vi "Power Output Execute Measurement.vi"(0 "Plots":T15, 1 "Measurement Data In":T11[](array[typedef]), 2 "TestSetDef":T1={"General"={"ID"=0, "Model"="", "Dual Port?"=FALSE, "Options"="", "Options"={"E"=FALSE, "K"=FALSE, "H"=FALSE, "W"=FALSE, "F"=FALSE}, "Cal File"=path ""}, "Receiver"={"Fstart, MHz"=0.0, "Fstop MHz"=0.0, "Fstep MHz"=0.0, "IF, MHz"=0.0}, "RX Band"={"Fstart, MHz"=0.0, "Fstop MHz"=0.0}, "TX 1"={"Fstart, MHz"=0.0, "Fstop MHz"=0.0, "Pmax, dBm"=0.0, "Pstep, dB"=0.0}, "TX 2"={"Fstart, MHz"=0.0, "Fstop MHz"=0.0, "Pmax, dBm"=0.0, "Pstep, dB"=0.0}, "Low-side?"=TRUE}, 3 "Queue":refnum<queue>, 5 "Test Parameters":T2={"Stimulus"={"Frequency Type"=enum."Band Edges", "Frequency Ranges"=[], "TX 1 Frequency (MHz)"={"Min"=0.0, "Max"=0.0}, "TX 2 Frequency (MHz)"={"Min"=0.0, "Max"=0.0}, "RX Frequency (MHz)"={"Min"=0.0, "Max"=0.0}, "Pad Model Number"="", "Pad Serial Number"="", "Pad Values"=[]}, "Measurement"={"DUT Port"=enum."Port 1", "Direction"=0, "Frequency Step Size"=0}, "Display"={"Frequency"={"Min"=-1.0, "Max"=-1.0}, "Power"={"Min"=-1, "Max"=-1}}, "Limit"={"Min Power (dBm)"=44.0}, "Calibration"={"Calibrated?"=FALSE}} {"Measurement"."Frequency Step Size" items=["0.2", "0.4", "1.0", "2.0", "4.0"]; "Measurement"."Direction" items=["Reverse", "Forward", "Auxiliary"]}, 9 "Measured Values":refnum<vi>, 11 "error in (no error)":errorcluster, 12 "Driver Refs In":T14, 13 "Measurements":refnum<vi>) -> (4 "Pass/Fail":bool[](array[boolean]), 6 "Test Parameters Out":T2={"Stimulus"={"Frequency Type"=enum."Band Edges", "Frequency Ranges"=[], "TX 1 Frequency (MHz)"={"Min"=0.0, "Max"=0.0}, "TX 2 Frequency (MHz)"={"Min"=0.0, "Max"=0.0}, "RX Frequency (MHz)"={"Min"=0.0, "Max"=0.0}, "Pad Model Number"="", "Pad Serial Number"="", "Pad Values"=[]}, "Measurement"={"DUT Port"=enum."Port 1", "Direction"=0, "Frequency Step Size"=0}, "Display"={"Frequency"={"Min"=-1.0, "Max"=-1.0}, "Power"={"Min"=-1, "Max"=-1}}, "Limit"={"Min Power (dBm)"=44.0}, "Calibration"={"Calibrated?"=FALSE}} {"Measurement"."Frequency Step Size" items=["0.2", "0.4", "1.0", "2.0", "4.0"]; "Measurement"."Direction" items=["Reverse", "Forward", "Auxiliary"]}, 10 "Measurement Data Out":T11[](array[typedef]), 14 "Driver Refs Out":T14, 15 "error out":errorcluster)   [LabVIEW 2011]
uses:
  TypeDefs/Power Output Test Parameters.ctl
  TypeDefs/Power Output Stimulus Parameters.ctl
  TypeDefs/Power Output Measurement Parameters.ctl
  BPIMCore EXT/HW IO/DUTport.ctl
  BPIMCore EXT/HW IO/MeasMode.ctl
  BPIMCore EXT/HW IO/PIM Sweep Step Size.ctl
  TypeDefs/Power Output Display Parameters.ctl
  TypeDefs/Power Output Limit Parameters.ctl
  TypeDefs/Power Output Calibration State.ctl
  drivers/PIM/PIM Driver Ref.ctl
  drivers/PWM/PWM Driver Ref.ctl
  TypeDefs/Power Output Measurement Data.ctl
  TypeDefs/Power Output Queue Cluster.ctl
  BPIMCore EXT/HW IO/Test Set Definition.ctl
  drivers/PIM/PIM Command.ctl
  Summitek EXT/Miscellaneous/OGAB Version.ctl
  drivers/PWM/PWM Parameters.ctl
  drivers/PWM/PWM Command.ctl
  Summitek EXT/OpenG EXT/array/array.llb/Remove Duplicates from 1D Array (DBL)__ogtk.vi
  <vilib>/Analysis/NI_AALBase.lvlib
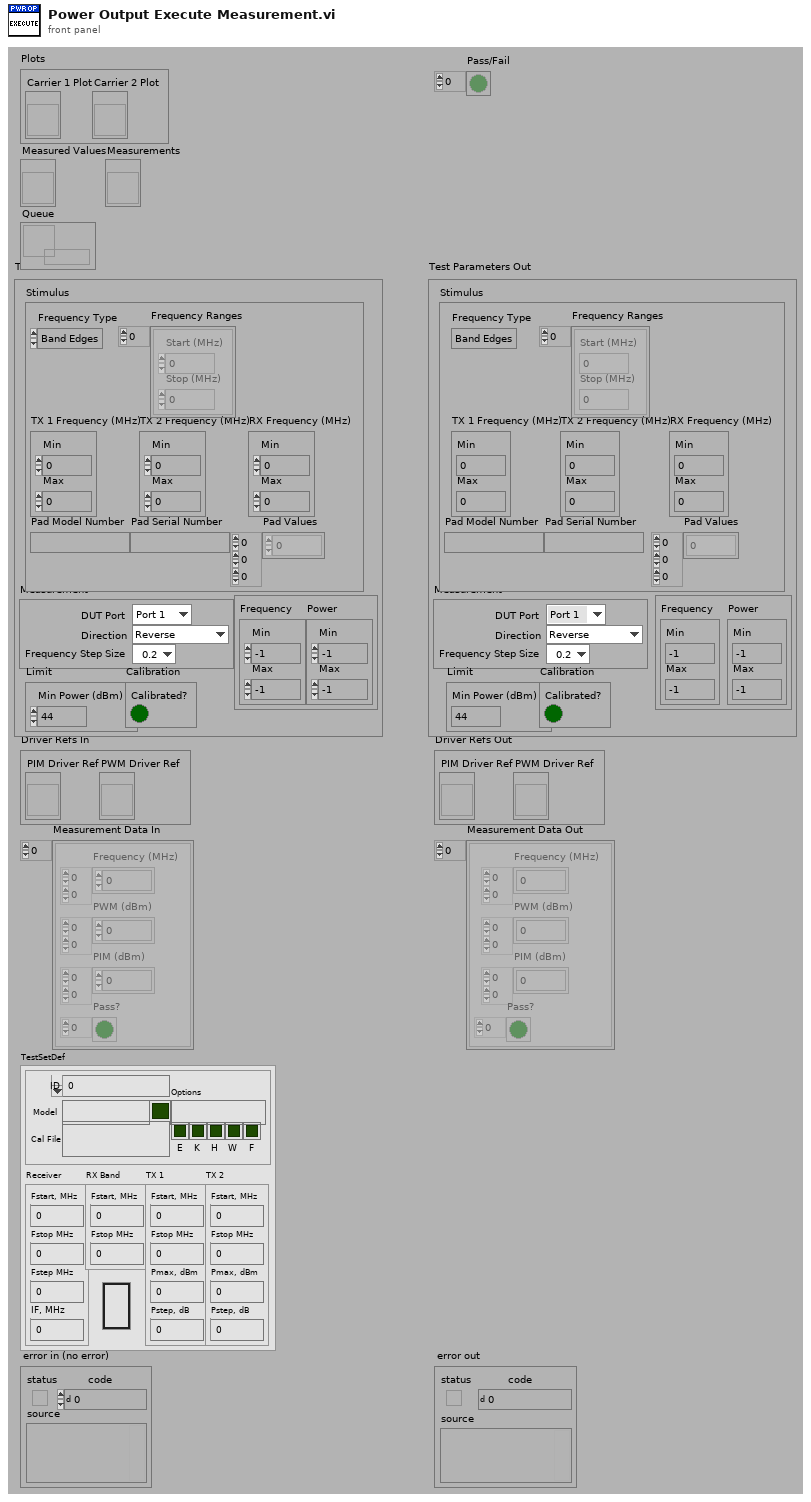
[diagram p1: front panel]
types:
  T1 = typedef "Test Set Definition.ctl" = cluster{"General":cluster{"ID":u32, "Model":string, "Dual Port?":bool, "Options":string, "Options":cluster{"E":bool, "K":bool, "H":bool, "W":bool, "F":bool}, "Cal File":path}, "Receiver":cluster{"Fstart, MHz":dbl, "Fstop MHz":dbl, "Fstep MHz":dbl, "IF, MHz":dbl}, "RX Band":cluster{"Fstart, MHz":dbl, "Fstop MHz":dbl}, "TX 1":cluster{"Fstart, MHz":dbl, "Fstop MHz":dbl, "Pmax, dBm":dbl, "Pstep, dB":dbl}, "TX 2":cluster{"Fstart, MHz":dbl, "Fstop MHz":dbl, "Pmax, dBm":dbl, "Pstep, dB":dbl}, "Low-side?":bool}
  T2 = typedef "Power Output Test Parameters.ctl" = cluster{"Stimulus":T3, "Measurement":T4, "Display":T8, "Limit":T9, "Calibration":T10}
  T3 = typedef "Power Output Stimulus Parameters.ctl" = cluster{"Frequency Type":enum16{"Band Edges", "Custom"}, "Frequency Ranges":cluster{"Start (MHz)":dbl, "Stop (MHz)":dbl}[], "TX 1 Frequency (MHz)":cluster{"Min":dbl, "Max":dbl}, "TX 2 Frequency (MHz)":cluster{"Min":dbl, "Max":dbl}, "RX Frequency (MHz)":cluster{"Min":dbl, "Max":dbl}, "Pad Model Number":string, "Pad Serial Number":string, "Pad Values":dbl[][][]}
  T4 = typedef "Power Output Measurement Parameters.ctl" = cluster{"DUT Port":T5, "Direction":T6, "Frequency Step Size":T7}
  T5 = typedef "DUTport.ctl" = enum16{"Port 1", "Port 2"}
  T6 = typedef "MeasMode.ctl" = u16
  T7 = typedef "PIM Sweep Step Size.ctl" = u16
  T8 = typedef "Power Output Display Parameters.ctl" = cluster{"Frequency":cluster{"Min":dbl, "Max":dbl}, "Power":cluster{"Min":i32, "Max":i32}}
  T9 = typedef "Power Output Limit Parameters.ctl" = cluster{"Min Power (dBm)":dbl}
  T10 = typedef "Power Output Calibration State.ctl" = cluster{"Calibrated?":bool}
  T11 = typedef "Power Output Measurement Data.ctl" = cluster{"Frequency (MHz)":dbl[][], "PWM (dBm)":dbl[][], "PIM (dBm)":dbl[][], "Pass?":bool[]}
  T12 = typedef "PIM Driver Ref.ctl" = refnum<vi>
  T13 = typedef "PWM Driver Ref.ctl" = refnum<vi>
  T14 = cluster{"PIM Driver Ref":T12, "PWM Driver Ref":T13}
  T15 = cluster{"Carrier 1 Plot":refnum<vi>, "Carrier 2 Plot":refnum<vi>}
  T16 = typedef "PIM Stimulus.ctl" = cluster{"Carrier Frequencies":cluster{"C1 Freq, MHz":dbl, "C2 Freq, MHz":dbl}, "Carrier Powers":cluster{"C1 Power,dBm":dbl, "C2 Power, dBm":dbl}, "Measurement Parameters":T17, "Measurement Setup":cluster{"Meas Type":enum32{"Time", "Frequency"}, "TXStep":T7}}
  T17 = typedef "PIM Cmd Params.ctl" = cluster{"IM Order":T18, "Averaging":T19, "Direction":T6, "Enable ALC?":bool, "Enable SingleIM?":bool, "Display Units":T20, "VA Hold?":bool, "DUT PORT":T5}
  T18 = typedef "IMOrder.ctl" = u8
  T19 = typedef "HW Averaging.ctl" = u16
  T20 = typedef "display_unit_format.ctl" = enum16{"dBm", "dBc"}
  T21 = typedef "PIM Command.ctl" = enum16{"LOAD", "KEEP ALIVE", "VALIDATE", "INITIALIZE", "PRESET", "GET CALIBRATION", "SET STIMULUS", "TOGGLE TX POWER", "SET TX ON", "SET TX OFF", "MEASURE", "UNLOAD"}
  T22 = typedef "OGAB Version.ctl" = cluster{"Version":string, "Build Number":u32, "Build Date/Time":dbl}
  T23 = typedef "PWM Parameters.ctl" = cluster{"Zero":bool, "Blank Screen":bool, "Offset":bool, "Offset Value":dbl, "Frequency (MHz)":dbl}
  T24 = typedef "PWM Command.ctl" = enum16{"LOAD", "INITIALIZE", "PRESET", "GET STIMULUS", "SET STIMULUS", "MEASURE", "RELEASE", "UNLOAD", "GET CALIBRATION", "CALIBRATE"}
  T25 = typedef "PWM Measurement.ctl" = dbl
  T26 = typedef "PIM Results.ctl" = cluster{"TxFreqs":dbl[], "TxPower":dbl[], "TxOn":bool[], "IMPower(s)":dbl[], "IMFreq(s)":dbl[], "Tx Stat":cluster{"CheckTx 1":bool, "Unlev Tx 1":bool, "Sql Tx 1":bool, "CheckTx 2":bool, "Unlev Tx 2":bool, "Sql Tx 2":bool}, "IM Overload":bool, "IMPower_dBc(s)":dbl[]}
  T27 = cluster{"duplicate driver ref":T12, "PWM Driver Ref":T13}
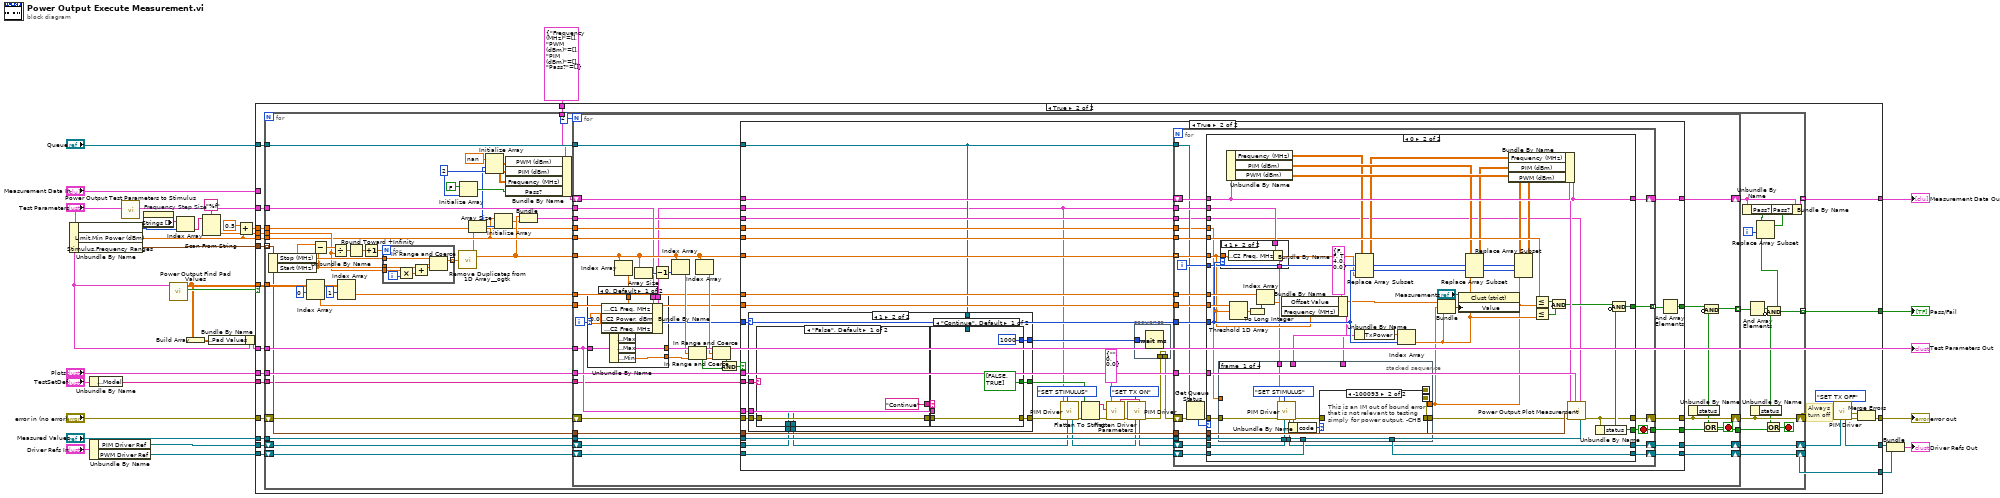
[diagram p0: block diagram]
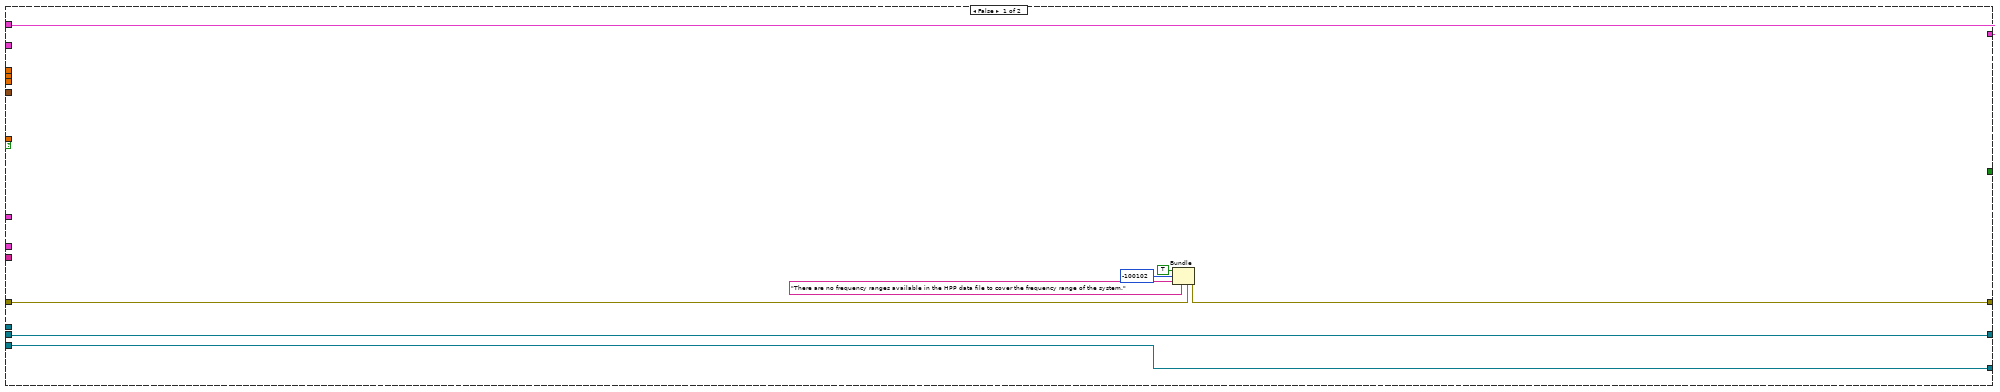
[diagram p2: hidden frame]
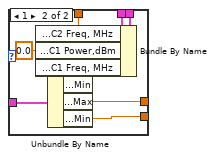
[diagram p3: hidden frame]
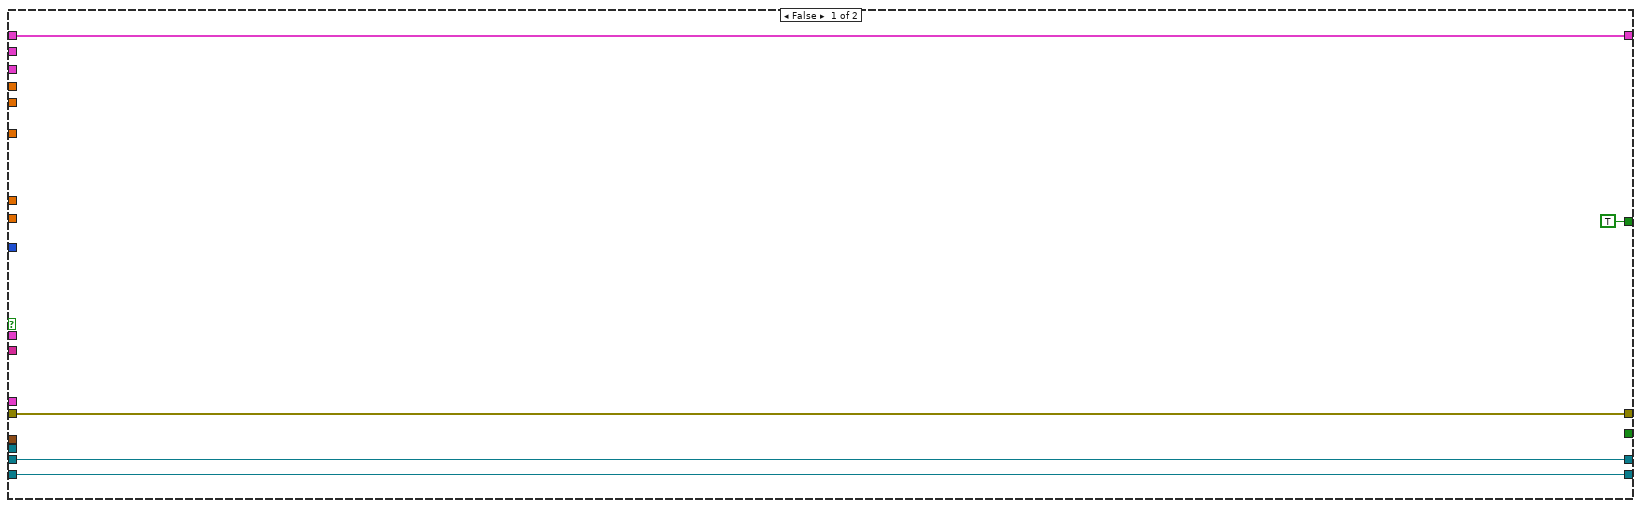
[diagram p4: hidden frame]
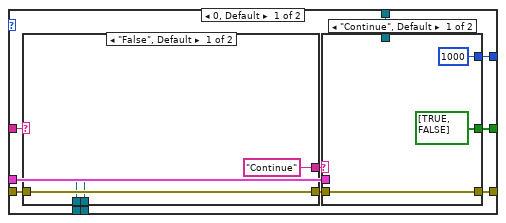
[diagram p5: hidden frame]
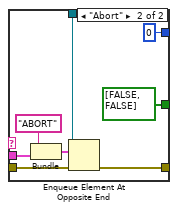
[diagram p6: hidden frame]
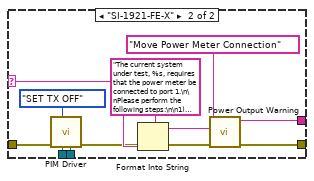
[diagram p7: hidden frame]
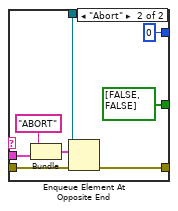
[diagram p8: hidden frame]
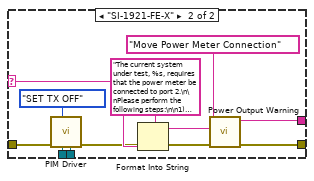
[diagram p9: hidden frame]
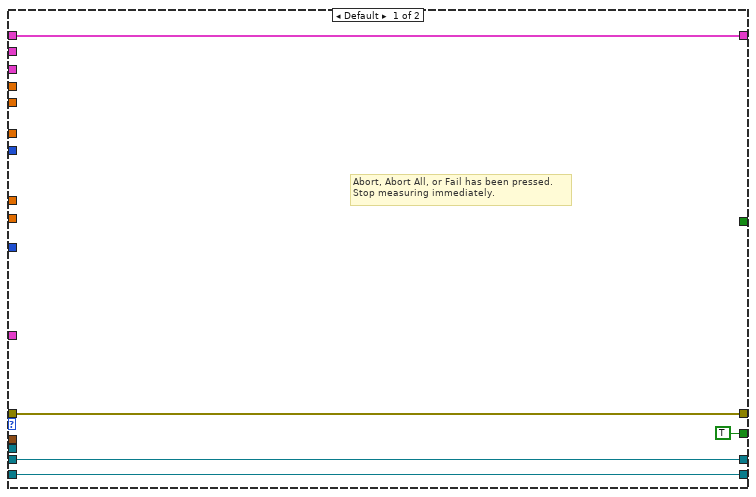
[diagram p10: hidden frame]
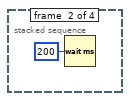
[diagram p12: hidden frame]
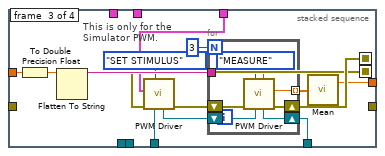
[diagram p13: hidden frame]
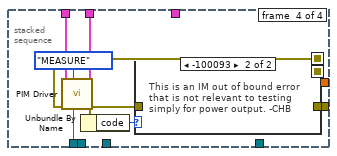
[diagram p14: hidden frame]
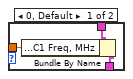
[diagram p16: hidden frame]
diagram:
  n1 = Unbundle By Name("Test Parameters") -> ("Measurement.Frequency Step Size"=w16:T7, "Limit.Min Power (dBm)"=w7:dbl, "Stimulus.Frequency Ranges"=w12:cluster{"Start (MHz)":dbl, "Stop (MHz)":dbl}[])
  n2 = Unbundle By Name("TestSetDef") -> ("General.Model"=w1:string)
  n3 = Unbundle By Name("Driver Refs In") -> ("PIM Driver Ref"=w27:T12, "PWM Driver Ref"=w28:T13)
  n4 = call "Power Output Test Parameters to Stimulus.vi"("PO Test Parameters"="Test Parameters") -> ("PIM Measurement Stimulus"=w31:T16)  [unwired: 10 out]
  n5 = property on="Frequency Step Size" class="Ring (strict)"() -> ("Strings []"=w17:string[])  [unwired: 2 in, 2 out]
  n6 = call "Power Output Find Pad Values.vi"("Test Parameters"="Test Parameters") -> ("Values Present?"=w24:bool, "Pad Values Out"=w10:dbl[][])  [unwired: 9 in]
  n7 = Index Array(array=w17, index=w16) -> (element=w15:string)
  n8 = Build Array(w10) -> (w9:dbl[][][])
  n9 = Scan From String(format string="%f", input string=w15) -> (output 1=w13:dbl)  [unwired: 3 in, 3 out]
  n10 = Bundle By Name(cluster="Test Parameters", "Stimulus.Pad Values"=w9) -> (w8:T2)
  "Test Parameters Out" <- w8
  n11 = Add(x=0.5 ("y"), y=w7) -> (x+y=w5:dbl)
  n12 = case shown="True" w24 {
    tunnel: w7 -> [_ w64]
    tunnel: w31 -> [_ w63]
    tunnel: [w38 w62] -> w30
    tunnel: [w36 w61] -> w29
    tunnel: w28 -> [w39 w58]
    tunnel: w27 -> [w40 w57]
    tunnel: "Plots" -> [_ w56]
    tunnel: "error in (no error)" -> [w37 w55]
    tunnel: w12 -> [_ w54]
    tunnel: w10 -> [_ w53]
    tunnel: [w40 w52] -> w22
    tunnel: [w39 w51] -> w21
    tunnel: "Measurement Data In" -> [w38 _]
    tunnel: w8 -> [_ w48]
    tunnel: "Measured Values" -> [_ w47]
    tunnel: [_ w46] -> w18
    tunnel: w13 -> [_ w45]
    tunnel: "Queue" -> [_ w44]
    tunnel: w5 -> [_ w43]
    tunnel: T11 {"Frequency (MHz)"=[], "PWM (dBm)"=[], "PIM (dBm)"=[], "Pass?"=[]} ("element") -> [_ w42]
    tunnel: w1 -> [_ w41]
    frame False {
      n13 = Bundle(cluster=w37, "status"=TRUE, "code"=-100102, "source"="There are no frequency ranges available in the HPP data file to cover the frequency range of the system.") -> (w36:errorcluster)
    }
    frame True {
      # "Always\nturn off"
      n14 = for {
        tunnel: w64 -> [w71]
        tunnel: w56 -> [w115]
        tunnel: w54 -> [w86] mode=indexing
        tunnel: w63 -> [w112]
        tunnel: w53 -> [w104]
        tunnel: [w76] -> w62 mode=indexing
        tunnel: [w73] -> w46 mode=indexing
        shift-right: [w105] -> w59
        shift-left: w55 -> [w113]
        shift-right: [w111] -> w60
        shift-left: w57 -> [w110]
        shift-right: [w114] -> w51
        shift-left: w58 -> [w109]
        tunnel: w48 -> [w100]
        tunnel: w47 -> [w99]
        tunnel: w45 -> [w92]
        tunnel: w44 -> [w85]
        tunnel: w43 -> [w67]
        tunnel: w42 -> [w66]
        tunnel: w41 -> [w65]
        i -> [w74]
        stop <- w82 stop-if-true
        w80 = 2 ("dimension size")
        n15 = Unbundle By Name(w86) -> ("Stop (MHz)"=w94:dbl, "Start (MHz)"=w93:dbl)
        n16 = Index Array(array=w104, index (row)=0 ("disabled index (col)")) -> (element=w90:dbl[])  [unwired: 1 in]
        n17 = Subtract(x=w94, y=w93) -> (x-y=w96:dbl)
        n18 = Divide(x=w96, y=w92) -> (x/y=w95:dbl)
        n19 = Index Array(array=w104, index (row)=1 ("disabled index (col)")) -> (element=w103:dbl[])  [unwired: 1 in]
        n20 = Round Toward +Infinity(x=w95) -> (ceil(x): smallest int >= x=w89:dbl)
        n21 = Increment(x=w89) -> (x+1=w88:dbl)
        n22 = for {
          N: w88 -> [_]
          tunnel: w94 -> [w118]
          tunnel: w93 -> [w119]
          tunnel: w92 -> [w122]
          tunnel: [w116] -> w87 mode=indexing
          i -> [w121]
          n23 = Multiply(x=w122, y=w121) -> (x*y=w120:dbl)
          n24 = Add(x=w119, y=w120) -> (x+y=w117:dbl)
          n25 = In Range and Coerce(upper limit=w118, x=w117, lower limit=w119) -> (coerced(x)=w116:dbl)  [unwired: 1 out]
        }
        n26 = call-poly "Remove Duplicates from 1D Array__ogtk.vi"("Input Array"=w87) -> ("Output Array"=w70:dbl[])  [unwired: 1 out]
        n27 = Initialize Array(FALSE ("Pass?"), w80) -> (w79:bool[])
        n28 = Array Size(array=w70) -> (size(s)=w72:i32)
        n29 = Initialize Array(nan ("Power (dBm)"), w72, w80) -> (w91:dbl[][])
        n30 = Initialize Array(w71, w72) -> (w69:dbl[])
        n31 = Bundle By Name(cluster=w66, "PWM (dBm)"=w91, "PIM (dBm)"=w91, "Frequency (MHz)"=w91, "Pass?"=w79) -> (w107:T11)
        n32 = Bundle("Output Array"=w70, w69) -> (w68:cluster{"Output Array":dbl[], dbl[]})  [unwired: 1 in]
        n33 = for {
          N: 2 -> [_]
          tunnel: w71 -> [w160]
          tunnel: w112 -> [w135]
          tunnel: w115 -> [w159]
          shift-right: [w155] -> w105
          shift-left: w113 -> [w126]
          shift-right: [w156] -> w111
          shift-left: w110 -> [w127]
          shift-right: [w157] -> w114
          shift-left: w109 -> [w158]
          tunnel: [w151] -> w98 mode=indexing
          shift-right: [w153] -> w77
          shift-left: w107 -> [w154]
          tunnel: w103 -> [w144]
          tunnel: w100 -> [w125]
          tunnel: w99 -> [w152]
          tunnel: w70 -> [w147]
          tunnel: w90 -> [w143]
          tunnel: w86 -> [w139]
          tunnel: w85 -> [w128]
          tunnel: [w137] -> w84
          tunnel: w68 -> [w130]
          tunnel: w67 -> [w129]
          tunnel: w65 -> [w124]
          i -> [w136]
          stop <- w138 stop-if-true
          n34 = Index Array(array=w147) -> (element=w134:dbl)  [unwired: 1 in]
          n35 = case shown="0, Default" w136 {
            tunnel: w135 -> [w168 w176]
            tunnel: w134 -> [w166 w174]
            tunnel: w125 -> [w162 w170]
            tunnel: [w164 w172] -> w133
            tunnel: [w163 w171] -> w132
            tunnel: [w161 w169] -> w123
            frame 0, Default {
              n36 = Unbundle By Name(w162) -> ("Stimulus.TX 2 Frequency (MHz).Max"=w165:dbl, "Stimulus.TX 1 Frequency (MHz).Max"=w164:dbl, "Stimulus.TX 1 Frequency (MHz).Min"=w163:dbl)
              n37 = Bundle By Name(cluster=w168, "Carrier Frequencies.C1 Freq, MHz"=w166, "Carrier Powers.C2 Power, dBm"=0.0, "Carrier Frequencies.C2 Freq, MHz"=w165) -> (w161:T16)
            }
            frame 1 {
              n38 = Unbundle By Name(w170) -> ("Stimulus.TX 1 Frequency (MHz).Min"=w173:dbl, "Stimulus.TX 2 Frequency (MHz).Max"=w172:dbl, "Stimulus.TX 2 Frequency (MHz).Min"=w171:dbl)
              n39 = Bundle By Name(cluster=w176, "Carrier Frequencies.C2 Freq, MHz"=w174, "Carrier Powers.C1 Power,dBm"=0.0, "Carrier Frequencies.C1 Freq, MHz"=w173) -> (w169:T16)
            }
          }
          n40 = Array Size(array=w147) -> (size(s)=w148:i32)
          n41 = Decrement(x=w148) -> (x-1=w142:i32)
          n42 = Index Array(array=w147, index=w142) -> (element=w145:dbl)
          n43 = In Range and Coerce(upper limit=w133, x=w145, lower limit=w132) -> (In Range?=w149:bool)  [unwired: 1 out]
          n44 = Index Array(array=w147) -> (element=w146:dbl)  [unwired: 1 in]
          n45 = In Range and Coerce(upper limit=w133, x=w146, lower limit=w132) -> (In Range?=w150:bool)  [unwired: 1 out]
          n46 = And(x=w150, y=w149) -> (x .and. y?=w141:bool)
          n47 = case shown="True" w141 {
            tunnel: w160 -> [_ w222]
            tunnel: w159 -> [_ w221]
            tunnel: w158 -> [w178 w220]
            tunnel: [w178 w219] -> w157
            tunnel: w127 -> [w179 w189]
            tunnel: w136 -> [_ w192]
            tunnel: [w179 w218] -> w156
            tunnel: [w180 w217] -> w155
            tunnel: w126 -> [w180 w191]
            tunnel: w154 -> [w181 w216]
            tunnel: [w181 w215] -> w153
            tunnel: w152 -> [_ w214]
            tunnel: w147 -> [_ w213]
            tunnel: w144 -> [_ w212]
            tunnel: w143 -> [_ w211]
            tunnel: w123 -> [_ w182]
            tunnel: [TRUE w209] -> w140
            tunnel: w139 -> [_ w208]
            tunnel: w128 -> [_ w187]
            tunnel: [_ w207] -> w137
            tunnel: w130 -> [_ w206]
            tunnel: w129 -> [_ w205]
            tunnel: w125 -> [_ w186]
            tunnel: w124 -> [_ w185]
            frame False {
            }
            frame True {
              n48 = case shown="1" w192 {
                tunnel: w191 -> [w233 w269]
                tunnel: [w232 w263] -> w190
                tunnel: w189 -> [w231 w268]
                tunnel: [w230 w267] -> w188
                tunnel: w187 -> [w229 w260]
                tunnel: w186 -> [w227 w265]
                tunnel: w185 -> [w226 w266]
                tunnel: [w225 w261] -> w184
                tunnel: [w224 w262] -> w183
                frame 0, Default {
                  n49 = case shown="\"False\", Default" w226 {
                    selector: w226 -> [_ w254]
                    tunnel: w233 -> [w247 w251]
                    tunnel: [w247 w257] -> w223
                    tunnel: ["Continue" ("Dialog Response") w253] -> w228
                    tunnel: w231 -> [w245 w250]
                    tunnel: [w245 w249] -> w230
                    frame "False", Default {
                    }
                    frame "SI-1921-FE-X" {
                      n50 = call "PIM Driver.vi"("Driver Ref (null)"=w250, "PIM Command"=PIM_Command."SET TX OFF", "error in (no error)"=w251) -> ("error out"=w248:errorcluster, "duplicate driver ref"=w249:T12)  [unwired: 2 in, 5 out]
                      n51 = Format Into String(format string="The current system under test, %s, requires that the power meter be connected to port 1.\n\nPlease perform the following steps:\n\n1)  Connect the Power Sensor to port 1;\n2)  Press Continue." ("F button name (\"Cancel\")"), w254) -> (resulting string=w255:string)  [unwired: 2 in, 1 out]
                      n52 = call "Power Output Warning.vi"("error in (no error)"=w248, "Message"=w255, "Header"="Move Power Meter Connection" ("F button name (\"Cancel\")")) -> ("error out"=w257:errorcluster, "Dialog Response"=w253:string)  [unwired: 7 in]
                    }
                  }
                  n53 = case shown="\"Continue\", Default" w228 {
                    tunnel: [bool[] [TRUE, FALSE] bool[] [FALSE, FALSE]] -> w224
                    tunnel: [u32 1000 ("milliseconds to wait") u32 0 ("milliseconds to wait")] -> w225
                    tunnel: w223 -> [w234 w242]
                    tunnel: [w234 w241] -> w232
                    tunnel: w229 -> [_ w238]
                    tunnel: w227 -> [_ w237]
                    frame "Continue", Default {
                    }
                    frame "Abort" {
                      n54 = Bundle("ABORT", "Test Parameters"=w237) -> (w239:cluster{string, "Test Parameters":T2})  [unwired: 1 out]
                      n55 = Enqueue Element At Opposite End(queue=w238, element=w239, error in (no error)=w242) -> (error out=w241:errorcluster)  [unwired: 1 in, 2 out]
                    }
                  }
                }
                frame 1 {
                  n56 = case shown="\"False\", Default" w266 {
                    selector: w266 -> [_ w290]
                    tunnel: w269 -> [w283 w287]
                    tunnel: [w283 w293] -> w259
                    tunnel: ["Continue" ("Dialog Response") w289] -> w264
                    tunnel: w268 -> [w281 w286]
                    tunnel: [w281 w285] -> w267
                    frame "False", Default {
                    }
                    frame "SI-1921-FE-X" {
                      n57 = call "PIM Driver.vi"("Driver Ref (null)"=w286, "PIM Command"=PIM_Command."SET TX OFF", "error in (no error)"=w287) -> ("error out"=w284:errorcluster, "duplicate driver ref"=w285:T12)  [unwired: 2 in, 5 out]
                      n58 = Format Into String(format string="The current system under test, %s, requires that the power meter be connected to port 2.\n\nPlease perform the following steps:\n\n1)  Connect the Power Sensor to port 2;\n2)  Press Continue." ("F button name (\"Cancel\")"), w290) -> (resulting string=w291:string)  [unwired: 2 in, 1 out]
                      n59 = call "Power Output Warning.vi"("error in (no error)"=w284, "Message"=w291, "Header"="Move Power Meter Connection" ("F button name (\"Cancel\")")) -> ("error out"=w293:errorcluster, "Dialog Response"=w289:string)  [unwired: 7 in]
                    }
                  }
                  n60 = case shown="\"Continue\", Default" w264 {
                    tunnel: [bool[] [FALSE, TRUE] bool[] [FALSE, FALSE]] -> w262
                    tunnel: [u32 1000 ("milliseconds to wait") u32 0 ("milliseconds to wait")] -> w261
                    tunnel: w259 -> [w270 w278]
                    tunnel: [w270 w277] -> w263
                    tunnel: w260 -> [_ w274]
                    tunnel: w265 -> [_ w273]
                    frame "Continue", Default {
                    }
                    frame "Abort" {
                      n61 = Bundle("ABORT", "Test Parameters"=w273) -> (w275:cluster{string, "Test Parameters":T2})  [unwired: 1 out]
                      n62 = Enqueue Element At Opposite End(queue=w274, element=w275, error in (no error)=w278) -> (error out=w277:errorcluster)  [unwired: 1 in, 2 out]
                    }
                  }
                }
              }
              n63 = call "PIM Driver.vi"("Driver Ref (null)"=w188, "PIM Command"=PIM_Command."SET STIMULUS", "error in (no error)"=w190, "Stimulus"=w182) -> ("error out"=w199:errorcluster, "duplicate driver ref"=w194:T12)  [unwired: 1 in, 5 out]
              n64 = Flatten To String(anything=w183, error in (no error)=w199) -> (data string=w203:string, error out=w198:errorcluster)  [unwired: 2 in, 1 out]
              n65 = call "Flatten Driver Parameters.vi"("error in (no error)"=w198, "Flattened Driver Parameters (\"\")"=w203, "Driver Version"=T22 {"Version"="", "Build Number"=0, "Build Date/Time"=0.0}) -> ("error out"=w197:errorcluster, "Flattened Driver Parameters with Version"=w204:string)  [unwired: 3 in]
              n66 = call "PIM Driver.vi"("PIM Driver Name/Configuration"=w204, "Driver Ref (null)"=w194, "PIM Command"=PIM_Command."SET TX ON", "error in (no error)"=w197) -> ("error out"=w202:errorcluster, "duplicate driver ref"=w193:T12)  [unwired: 1 in, 5 out]
              n67 = stacked-sequence {
                tunnel: w202 -> [w296]
                tunnel: [w296] -> w196
                tunnel: w184 -> [w295]
                frame #0 {
                  n68 = Wait (ms)(milliseconds to wait=w295) -> ()  [unwired: 1 out]
                }
              }
              n69 = for {
                tunnel: w182 -> [w320]
                tunnel: [w321] -> w210 mode=indexing
                tunnel: w221 -> [w314]
                shift-right: [w308] -> w219
                shift-left: w220 -> [w319]
                shift-right: [w309] -> w218
                shift-left: w193 -> [w318]
                tunnel: w222 -> [w312]
                shift-right: [w313] -> w215
                shift-left: w216 -> [w316]
                shift-right: [w310] -> w217
                shift-left: w196 -> [w303]
                tunnel: w212 -> [w317]
                tunnel: w192 -> [w315]
                tunnel: w214 -> [w307]
                tunnel: w213 -> [w306] mode=indexing
                tunnel: w211 -> [w305]
                tunnel: w208 -> [w304]
                tunnel: w187 -> [w301]
                tunnel: [w299] -> w207
                tunnel: w206 -> [w298]
                tunnel: w205 -> [w297]
                i -> [w311]
                stop <- w299 stop-if-true
                n70 = Get Queue Status(queue=w301, error in (no error)=w303) -> (error out=w302:errorcluster, # elements in queue=w300:i32)  [unwired: 1 in, 6 out]
                n71 = case shown="0" w300 {
                  tunnel: [_ w370] -> w321
                  tunnel: w320 -> [_ w369]
                  tunnel: w319 -> [w323 w338]
                  tunnel: w318 -> [w324 w339]
                  tunnel: w317 -> [_ w368]
                  tunnel: w316 -> [w326 w367]
                  tunnel: w315 -> [_ w346]
                  tunnel: w314 -> [_ w366]
                  tunnel: [w326 w365] -> w313
                  tunnel: w312 -> [_ w364]
                  tunnel: w311 -> [_ w344]
                  tunnel: [TRUE ("status") w362] -> w299
                  tunnel: [w325 w361] -> w310
                  tunnel: [w324 w336] -> w309
                  tunnel: [w323 w337] -> w308
                  tunnel: w307 -> [_ w360]
                  tunnel: w306 -> [_ w342]
                  tunnel: w305 -> [_ w359]
                  tunnel: w304 -> [_ w348]
                  tunnel: w302 -> [w325 w341]
                  tunnel: w298 -> [_ w343]
                  tunnel: w297 -> [_ w332]
                  frame Default {
                    # "Abort, Abort All, or Fail has been pressed.\nStop measuring immediately."
                  }
                  frame 0 {
                    n72 = case shown="1" w346 {
                      tunnel: w369 -> [w413 w416]
                      tunnel: w342 -> [w412 w415]
                      tunnel: [w411 w414] -> w334
                      frame 0, Default {
                        n73 = Bundle By Name(cluster=w413, "Carrier Frequencies.C1 Freq, MHz"=w412) -> (w411:T16)
                      }
                      frame 1 {
                        n74 = Bundle By Name(cluster=w416, "Carrier Frequencies.C2 Freq, MHz"=w415) -> (w414:T16)
                      }
                    }
                    n75 = Unbundle By Name(w367) -> ("Frequency (MHz)"=w354:dbl[][], "PIM (dBm)"=w356:dbl[][], "PWM (dBm)"=w357:dbl[][])
                    n76 = Threshold 1D Array(2:w342, 3:w359) -> (0:w349:dbl)  [unwired: 1 out]
                    n77 = To Long Integer(number=w349) -> (32bit integer=w350:i32)
                    n78 = Index Array(array=w368, index=w350) -> (element=w327:dbl)
                    n79 = Bundle By Name(cluster=T23 {"Zero"=FALSE, "Blank Screen"=FALSE, "Offset"=TRUE, "Offset Value"=4.0, "Frequency (MHz)"=0.0} ("PWM Stimulus"), "Offset Value"=w327, "Frequency (MHz)"=w342) -> (w333:T23)
                    n80 = stacked-sequence {
                      seq-local: [w372 _ _ _] -> [_ _ w385 _]
                      seq-local: [_ _ w393 _] -> [_ _ _ w402]
                      tunnel: [w377 _ _ _] -> w336
                      tunnel: [_ _ _ w404] -> w335
                      tunnel: w334 -> [w376 _ _ w406]
                      tunnel: w339 -> [w375 _ _ w407]
                      tunnel: w341 -> [w374 _ _ _]
                      tunnel: [_ _ _ w403] -> w340
                      tunnel: [_ _ w387 _] -> w337
                      tunnel: [_ _ w391 _] -> w328
                      tunnel: w338 -> [_ _ w383 _]
                      tunnel: w332 -> [_ _ w389 _]
                      tunnel: w333 -> [_ _ w381 _]
                      frame #0 {
                        n81 = call "PIM Driver.vi"("Driver Ref (null)"=w375, "PIM Command"=PIM_Command."SET STIMULUS", "error in (no error)"=w374, "Stimulus"=w376) -> ("error out"=w373:errorcluster, "duplicate driver ref"=w377:T12)  [unwired: 1 in, 5 out]
                        n82 = Unbundle By Name(w373) -> ("code"=w371:i32)
                        n83 = case shown="-100093" w371 {
                          tunnel: w373 -> [w379 _]
                          tunnel: [w379 _] -> w372
                          frame Default {
                          }
                          frame -100093 {
                            # "This is an IM out of bound error\nthat is not relevant to testing\nsimply for power output. -CHB"
                          }
                        }
                      }
                      frame #1 {
                        n84 = Wait (ms)(milliseconds to wait=u32 200) -> ()  [unwired: 1 out]
                      }
                      frame #2 {
                        # "This is only for the\nSimulator PWM."
                        n85 = To Double Precision Float(number=w389) -> (double precision float=w388:dbl)
                        n86 = Flatten To String(anything=w388) -> (data string=w390:string)  [unwired: 3 in, 2 out]
                        n87 = call "PWM Driver.vi"("Drv Refnum"=w383, "PWM Command"=PWM_Command."SET STIMULUS", "error in (no error)"=w385, "PWM Stimulus"=w381) -> ("error out"=w384:errorcluster, "dup Drv Refnum"=w382:T13)  [unwired: 4 in, 2 out]
                        n88 = for {
                          N: 3 -> [_]
                          tunnel: [w398] -> w392 mode=indexing
                          shift-right: [w400] -> w393
                          shift-left: w384 -> [w399]
                          tunnel: w390 -> [w396]
                          shift-right: [w395] -> w387
                          shift-left: w382 -> [w397]
                          n89 = call "PWM Driver.vi"("PWM Configuration (\"\")"=w396, "Drv Refnum"=w397, "PWM Command"=PWM_Command."MEASURE", "error in (no error)"=w399) -> ("error out"=w400:errorcluster, "PWM Measurement"=w398:T25, "dup Drv Refnum"=w395:T13)  [unwired: 4 in, 1 out]
                        }
                        n90 = call <vilib>:"Mean.vi"("X"=w392) -> ("mean"=w391:dbl)  [unwired: 1 out]
                      }
                      frame #3 {
                        n91 = call "PIM Driver.vi"("Driver Ref (null)"=w407, "PIM Command"=PIM_Command."MEASURE", "error in (no error)"=w402, "Stimulus"=w406) -> ("error out"=w405:errorcluster, "Measurement Results"=w404:T26)  [unwired: 1 in, 5 out]
                        n92 = Unbundle By Name(w405) -> ("code"=w409:i32)
                        n93 = case shown="-100093" w409 {
                          tunnel: w405 -> [w410 _]
                          tunnel: [w410 _] -> w403
                          frame Default {
                          }
                          frame -100093 {
                            # "This is an IM out of bound error\nthat is not relevant to testing\nsimply for power output. -CHB"
                          }
                        }
                      }
                    }
                    n94 = Unbundle By Name(w335) -> ("TxPower"=w358:dbl[])
                    n95 = Replace Array Subset(array=w354, new element=w342, index (row)=w344, index (col)=w346) -> (w353:dbl[][])
                    n96 = Index Array(array=w358, index=w346) -> (element=w329:dbl)
                    n97 = Bundle("Numeric"=w327, "mean"=w328, w329) -> (w331:cluster{"Numeric":dbl, "mean":dbl, dbl})  [unwired: 1 in]
                    n98 = property class="Clust (strict)"(reference="Measurements", "Value"=w331) -> ()  [unwired: 1 in, 2 out]
                    n99 = Replace Array Subset(array=w356, new element=w329, index (row)=w344, index (col)=w346) -> (w355:dbl[][])
                    n100 = Replace Array Subset(array=w357, new element=w328, index (row)=w344, index (col)=w346) -> (w345:dbl[][])
                    n101 = Bundle By Name(cluster=w367, "Frequency (MHz)"=w353, "PIM (dBm)"=w355, "PWM (dBm)"=w345) -> (w365:T11)
                    n102 = Less Or Equal?(x=w364, y=w328) -> (x <= y?=w352:bool)
                    n103 = Less Or Equal?(x=w364, y=w329) -> (x <= y?=w351:bool)
                    n104 = And(x=w352, y=w351) -> (x .and. y?=w363:bool)
                    n105 = call "Power Output Plot Measurement.vi"("Measured Values"=w360, "Minimum Power"=w343, "Plots"=w366, "error in (no error)"=w340, "Frequency Range (MHz)"=w348, "Measurement Data"=w365) -> ("error out"=w361:errorcluster)  [unwired: 5 in]
                    n106 = Unbundle By Name(w361) -> ("status"=w362:bool)
                    n107 = Compound Arithmetic op=AND(w363, invert w362) -> (w370:bool)
                  }
                }
              }
              n108 = And Array Elements(Boolean array=w210) -> (logical AND=w209:bool)
            }
          }
          n109 = Unbundle By Name(w155) -> ("status"=w131:bool)
          n110 = Or(x=w131, y=w137) -> (x .or. y?=w138:bool)
          n111 = Compound Arithmetic op=AND(w140, invert w131) -> (w151:bool)
        }
        n112 = Unbundle By Name(w77) -> ("Pass?"=w78:bool[])
        n113 = And Array Elements(Boolean array=w98) -> (logical AND=w97:bool)
        n114 = Unbundle By Name(w105) -> ("status"=w83:bool)
        n115 = Or(x=w83, y=w84) -> (x .or. y?=w82:bool)
        n116 = Compound Arithmetic op=AND(w97, invert w83) -> (w73:bool)
        n117 = Replace Array Subset(array=w78, new element=w73, index=w74) -> (w75:bool[])
        n118 = Bundle By Name(cluster=w77, "Pass?"=w75) -> (w76:T11)
      }
      n119 = call "PIM Driver.vi"("Driver Ref (null)"=w60, "PIM Command"=PIM_Command."SET TX OFF") -> ("error out"=w49:errorcluster, "duplicate driver ref"=w52:T12)  [unwired: 3 in, 5 out]
      n120 = Merge Errors(w59, w49) -> (w61:errorcluster)
    }
  }
  "error out" <- w29
  "Pass/Fail" <- w18
  "Measurement Data Out" <- w30
  n121 = Bundle("duplicate driver ref"=w22, "PWM Driver Ref"=w21) -> (→"Driver Refs Out":T27)  [unwired: 1 in]
